vi "vectorCalc.vi"(9 "b":cluster{"xPos":dbl, "yPos":dbl, "Theta":dbl}={"xPos"=1422.7656630990646, "yPos"=3772.073115389546, "Theta"=-70.44310923754139}, 10 "a":cluster{"xPos":dbl, "yPos":dbl, "Theta":dbl}={"xPos"=1422.7656630990646, "yPos"=3772.073115389546, "Theta"=-70.44310923754139}) -> (2 "a +/- b":cluster{"xPos":dbl, "yPos":dbl, "Theta":dbl})   [LabVIEW 2016]
panel:
  in  "operator":u16(ring) items=["Subtract", "Add"]
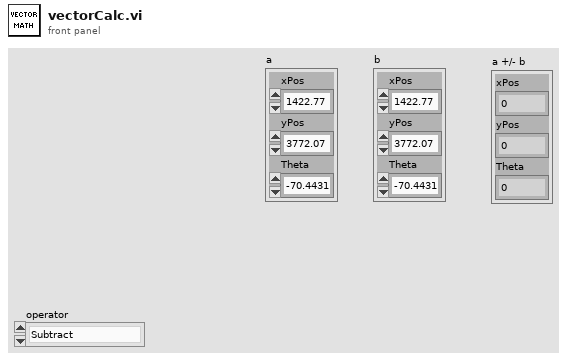
[diagram p1: front panel]
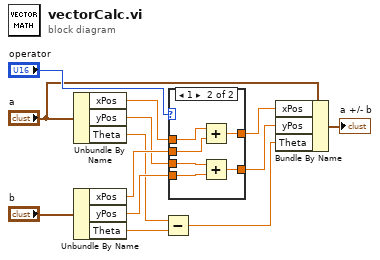
[diagram p0: block diagram]
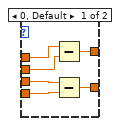
[diagram p2: hidden frame]
diagram:
  n1 = Unbundle By Name("a") -> ("xPos"=w11:dbl, "yPos"=w9:dbl, "Theta"=w4:dbl)
  n2 = Unbundle By Name("b") -> ("xPos"=w10:dbl, "yPos"=w8:dbl, "Theta"=w3:dbl)
  n3 = Subtract(x=w4, y=w3) -> (x-y=w2:dbl)
  n4 = case shown="1" "operator" {
    tunnel: w11 -> [w19 w25]
    tunnel: w10 -> [w18 w24]
    tunnel: w9 -> [w17 w23]
    tunnel: w8 -> [w16 w22]
    tunnel: [w15 w21] -> w6
    tunnel: [w14 w20] -> w5
    frame 0, Default {
      n5 = Subtract(x=w19, y=w18) -> (x-y=w15:dbl)
      n6 = Subtract(x=w17, y=w16) -> (x-y=w14:dbl)
    }
    frame 1 {
      n7 = Add(x=w25, y=w24) -> (x+y=w21:dbl)
      n8 = Add(x=w23, y=w22) -> (x+y=w20:dbl)
    }
  }
  n9 = Bundle By Name(cluster="a", "xPos"=w6, "yPos"=w5, "Theta"=w2) -> (→"a +/- b":cluster{"xPos":dbl, "yPos":dbl, "Theta":dbl})
